vi "FeedbackDecode_Str2Array.vi"(3 "StringIn":string) -> (0 "ArrayOut":dbl[][](array[numeric]), 1 "StrArrayOut":string[][](array[string]))   [LabVIEW 2020]
uses:
  <vilib>/regexp/Match Regular Expression.xnode
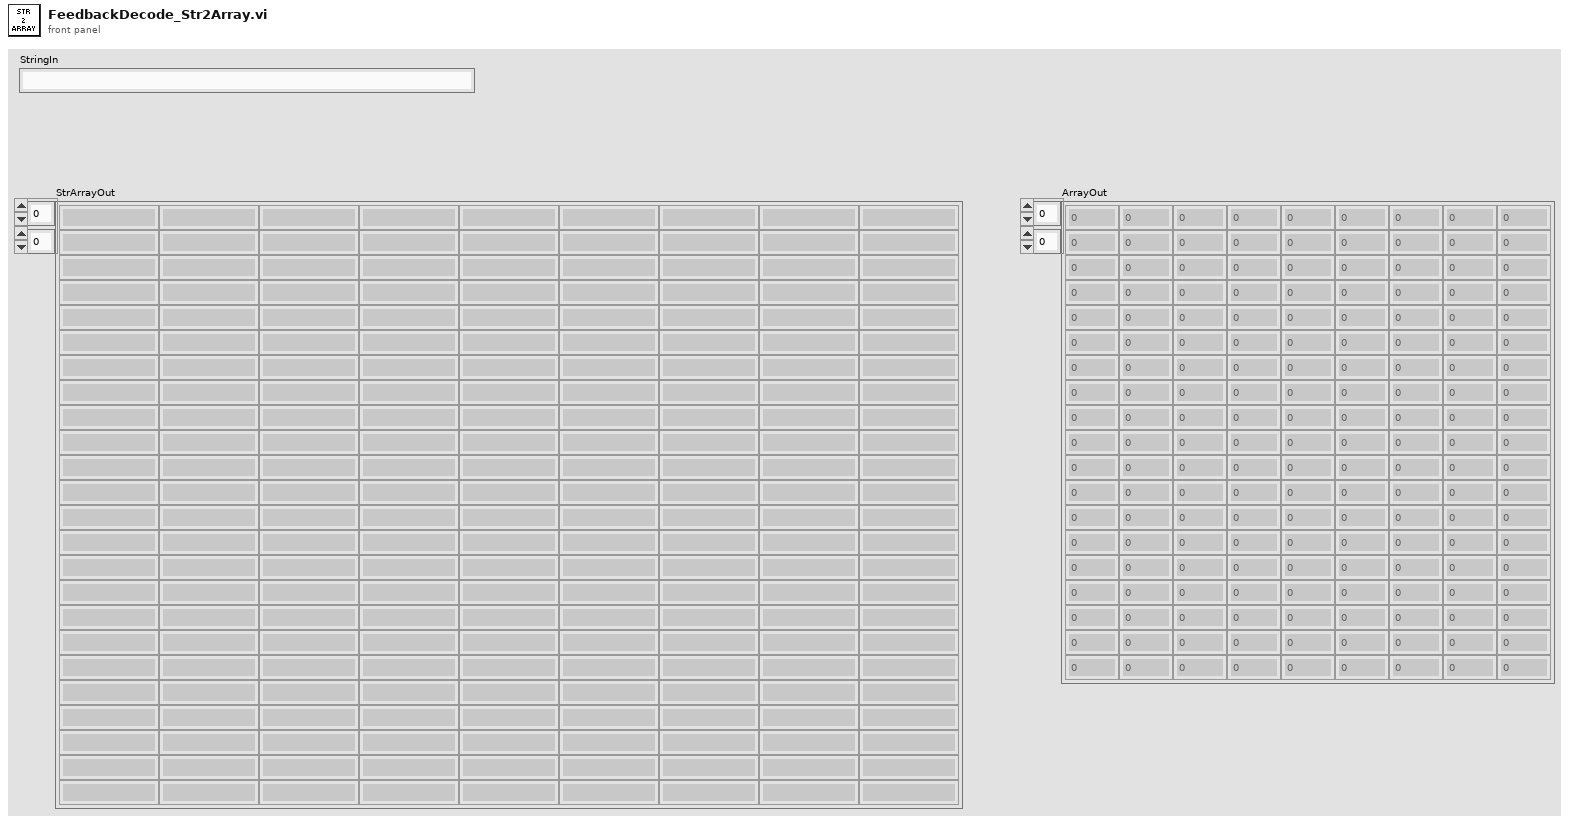
[diagram p1: front panel]
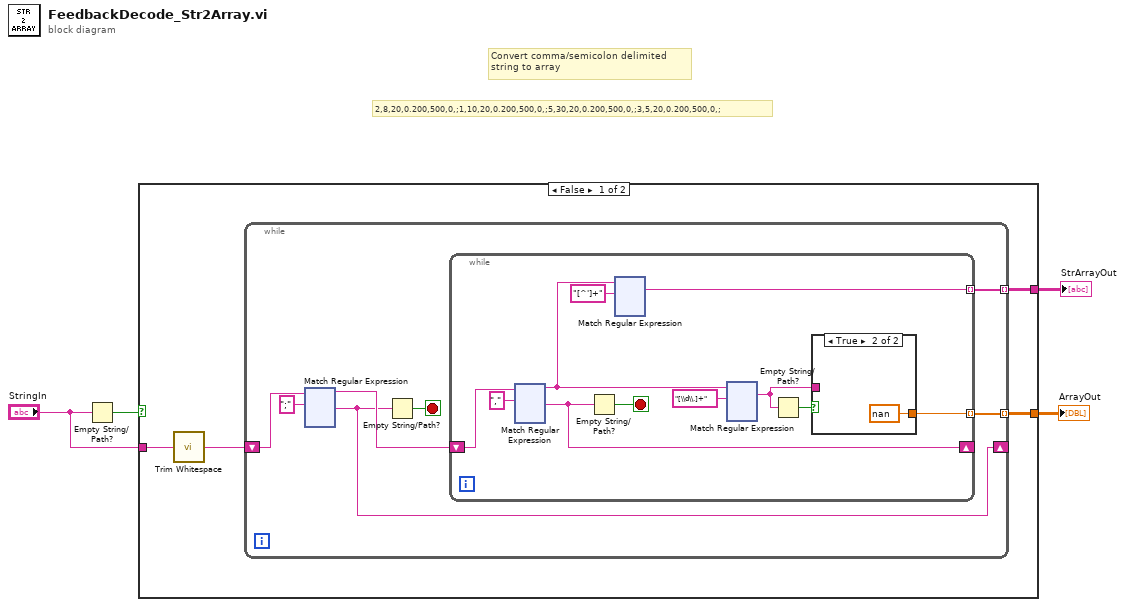
[diagram p0: block diagram]
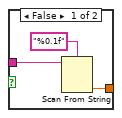
[diagram p2: hidden frame]
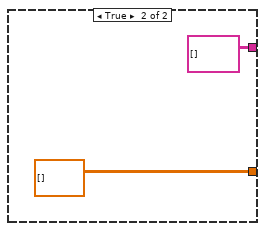
[diagram p3: hidden frame]
diagram:
  # "Convert comma/semicolon delimited\nstring to array"
  # "2,8,20,0.200,500,0,;1,10,20,0.200,500,0,;5,30,20,0.200,500,0,;3,5,20,0.200,500,0,;"
  n1 = Empty String/Path?(string/path="StringIn") -> (empty?=w4:bool)
  n2 = case shown="False" w4 {
    tunnel: "StringIn" -> [w8 _]
    tunnel: [w6 dbl[][] []] -> w3
    tunnel: [w5 string[][] []] -> w1
    frame False {
      n3 = call <vilib>:"Trim Whitespace.vi"("string"=w8) -> ("trimmed string"=w7:string)  [unwired: 1 in]
      n4 = while {
        tunnel: [w15] -> w6 mode=indexing
        shift-right: [w10] -> _
        shift-left: w7 -> [w13]
        tunnel: [w9] -> w5 mode=indexing
        stop <- w12 stop-if-true
        n5 = xnode "Match Regular Expression"("input string"=w13, "regular expression"=";") -> ("before match"=w11:string, "after match"=w10:string)  [unwired: 4 in, 3 out]
        n6 = Empty String/Path?(string/path=w10) -> (empty?=w12:bool)
        n7 = while {
          shift-right: [w134] -> _
          shift-left: w11 -> [w136]
          tunnel: [w135] -> w15 mode=indexing
          tunnel: [w127] -> w9 mode=indexing
          stop <- w133 stop-if-true
          n8 = xnode "Match Regular Expression"("input string"=w136, "regular expression"=",") -> ("before match"=w128:string, "after match"=w134:string)  [unwired: 4 in, 3 out]
          n9 = Empty String/Path?(string/path=w134) -> (empty?=w133:bool)
          n10 = xnode "Match Regular Expression"("input string"=w128, "regular expression"="[^']+") -> ("whole match"=w127:string)  [unwired: 4 in, 4 out]
          n11 = xnode "Match Regular Expression"("input string"=w128, "regular expression"="[\\d\\.]+") -> ("whole match"=w130:string)  [unwired: 4 in, 4 out]
          n12 = Empty String/Path?(string/path=w130) -> (empty?=w131:bool)
          n13 = case shown="True" w131 {
            tunnel: [w254 nan] -> w135
            tunnel: w130 -> [w252 _]
            frame False {
              n14 = Scan From String(format string="%0.1f", input string=w252) -> (output 1=w254:dbl)  [unwired: 3 in, 3 out]
            }
            frame True {
            }
          }
        }
      }
    }
    frame True {
    }
  }
  "ArrayOut" <- w3
  "StrArrayOut" <- w1
